vi "读取-缓存数据文件夹至报警记录列表.vi"() -> (0 "文件名":string[](array[string]), 1 "新记录文件名":string[](array[string]), 2 "新记录列表":string[][](array[string]), 3 "报警记录列表":string[][](array[string]))   [LabVIEW 2017]
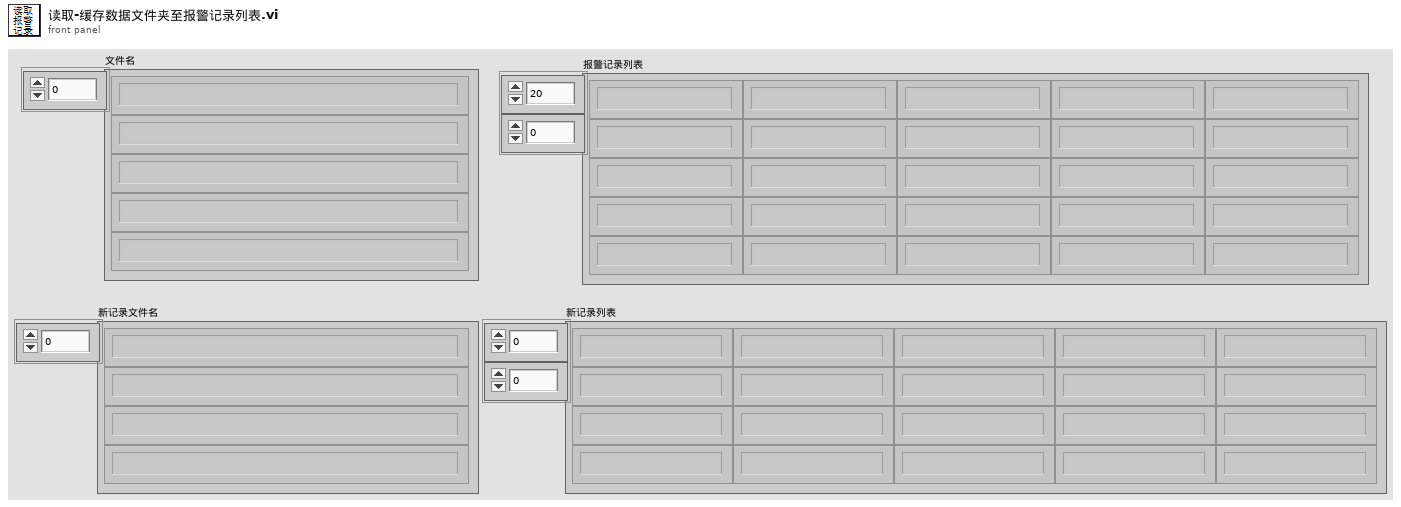
[diagram p1: front panel]
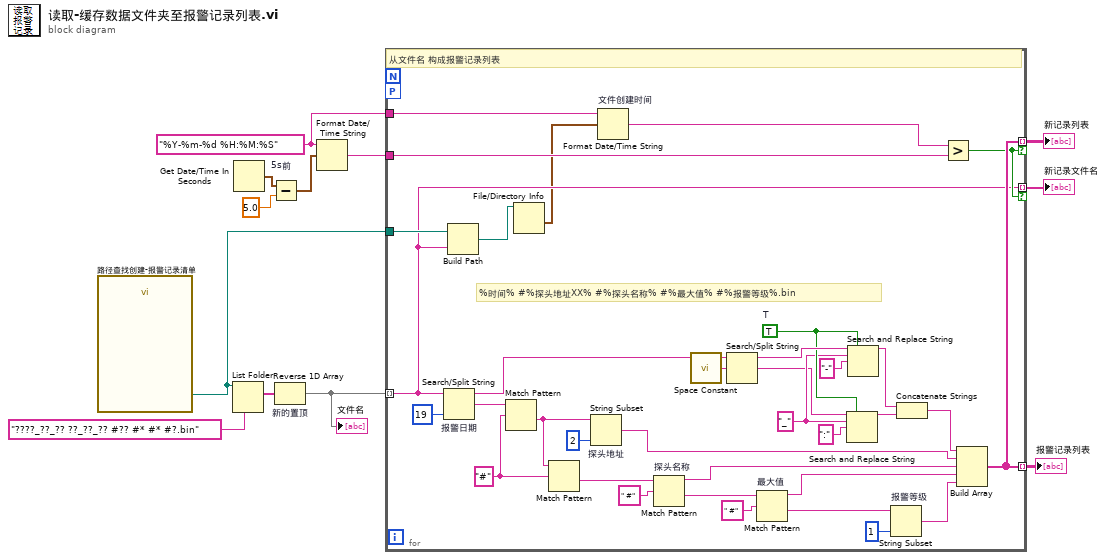
[diagram p0: block diagram]
diagram:
  w2 = "%Y-%m-%d %H:%M:%S" ("时间格式字符串(%c)")
  n1 = call "路径查找创建-报警记录清单.vi"() -> ("缓存数据文件夹"=w1:path)  [unwired: 8 in, 11 out]
  n2 = List Folder(path=w1, pattern="????_??_?? ??_??_?? #?? #* #* #?.bin" ("模式")) -> (filenames=w11:string[])  [unwired: 2 in, 3 out]
  n3 = Get Date/Time In Seconds() -> (seconds since 1Jan1904=w8:timestamp)
  n4 = Subtract "5s前"(x=w8, y=5.0) -> (x-y=w6:timestamp)
  n5 = Reverse 1D Array "新的置顶"(array=w11) -> (reversed array=w9:string[])
  "文件名" <- w9
  n6 = Format Date/Time String(time format string (%c)=w2, seconds (now)=w6) -> (date/time string=w5:string)  [unwired: 1 in]
  n7 = for {
    tunnel: w9 -> [w15] mode=indexing
    tunnel: [w20] -> w10 mode=indexing
    tunnel: w5 -> [w22]
    tunnel: [w20] -> w4 mode=indexing if=w19
    tunnel: [w15] -> w3 mode=indexing if=w19
    tunnel: w2 -> [w18]
    tunnel: w1 -> [w16]
    workers-P: _ -> [_]
    w28 = "_" ("搜索字符串")
    w29 = TRUE  # T
    w39 = "#" ("正则表达式")
    # "%时间% #%探头地址XX% #%探头名称% #%最大值% #%报警等级%.bin"
    # "从文件名 构成报警记录列表"
    n8 = Search/Split String "报警日期"(string=w15, offset (0)=19 ("偏移量(0)")) -> (substring before match=w32:string, match + rest of string=w46:string)  [unwired: 1 in, 1 out]
    n9 = Build Path(base path=w16, name or relative path=w15) -> (appended path=w17:path)
    n10 = Match Pattern(string=w46, regular expression=w39) -> (after substring=w44:string)  [unwired: 1 in, 3 out]
    n11 = File/Directory Info(path=w17) -> (last mod=w14:timestamp)  [unwired: 1 in, 6 out]
    n12 = Match Pattern(string=w44, regular expression=w39) -> (after substring=w37:string)  [unwired: 1 in, 3 out]
    n13 = String Subset "探头地址"(string=w44, length (rest)=2 ("长度（剩余）")) -> (substring=w42:string)  [unwired: 1 in]
    n14 = Format Date/Time String "文件创建时间"(time format string (%c)=w18, seconds (now)=w14) -> (date/time string=w13:string)  [unwired: 1 in]
    n15 = Match Pattern "探头名称"(string=w37, regular expression=" #" ("正则表达式")) -> (before substring=w33:string, after substring=w36:string)  [unwired: 1 in, 2 out]
    n16 = call <vilib>:"Space Constant.vi"() -> ("String"=w31:string)
    n17 = Search/Split String(string=w32, search string/char (-)=w31) -> (substring before match=w30:string, match + rest of string=w27:string)  [unwired: 1 in, 1 out]
    n18 = Match Pattern "最大值"(string=w36, regular expression=" #" ("正则表达式")) -> (before substring=w34:string, after substring=w40:string)  [unwired: 1 in, 2 out]
    n19 = Search and Replace String(replace all?=w29, input string=w27, search string=w28, replace string=":" ("搜索字符串")) -> (result string=w23:string)  [unwired: 4 in, 3 out]
    n20 = Search and Replace String(replace all?=w29, input string=w30, search string=w28, replace string="-" ("搜索字符串")) -> (result string=w24:string)  [unwired: 4 in, 3 out]
    n21 = String Subset "报警等级"(string=w40, length (rest)=1 ("长度（剩余）")) -> (substring=w35:string)  [unwired: 1 in]
    n22 = Concatenate Strings(w24, w23) -> (w21:string)
    n23 = Greater?(x=w13, y=w22) -> (0:w19:bool)
    n24 = Build Array(w21, w42, w33, w34, w35) -> (w20:string[])
  }
  "报警记录列表" <- w10
  "新记录列表" <- w4
  "新记录文件名" <- w3
